vi "Get Hand Info.vi"(10 "Bid":u64, 11 "Hand":string) -> (3 "Hand Info":T1)   [LabVIEW 2023, in "d7.lvlib"]
uses:
  d7.lvlib
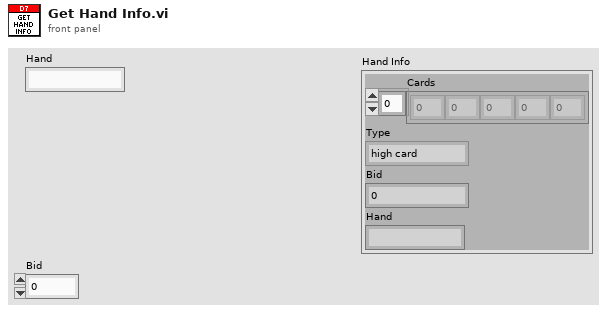
[diagram p1: front panel]
types:
  T1 = cluster{"Cards":i32[], "Type":enum16{"high card", "pair", "two pair", "3 of a kind", "full house", "4 of a kind", "5 of a kind"}, "Bid":u64, "Hand":string}
  T2 = enum16{"high card", "pair", "two pair", "3 of a kind", "full house", "4 of a kind", "5 of a kind"}
  T3 = cluster{i32[], enum16{"high card", "pair", "two pair", "3 of a kind", "full house", "4 of a kind", "5 of a kind"}, "Bid":u64, "Hand":string}
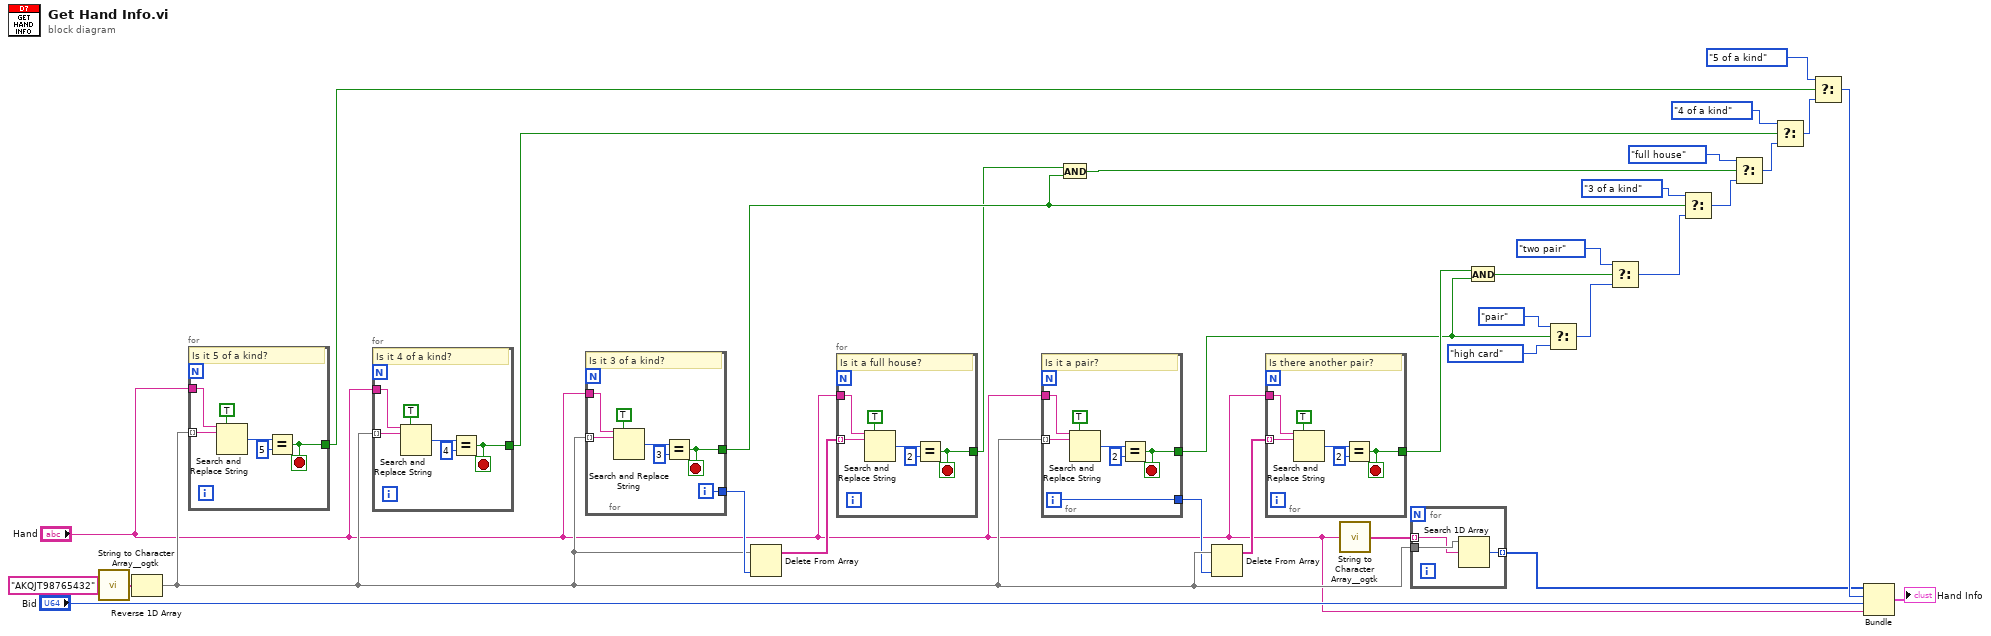
[diagram p0: block diagram]
diagram:
  n1 = call <userlib>:"String to Character Array__ogtk.vi"("Input String"="AKQJT98765432" ("regular expression")) -> ("Character Array"=w17:string[])
  n2 = Reverse 1D Array(array=w17) -> (reversed array=w16:string[])
  n3 = for {
    tunnel: w16 -> [w38] mode=indexing
    tunnel: "Hand" -> [w39]
    tunnel: [w34] -> w31
    stop <- w34 stop-if-true
    # "Is it 5 of a kind?"
    n4 = Search and Replace String(replace all?=TRUE ("replace all? (F)"), input string=w39, search string=w38) -> (number of replacements=w36:i32)  [unwired: 5 in, 3 out]
    n5 = Equal?(x=w36, y=5) -> (x = y?=w34:bool)
  }
  n6 = for {
    tunnel: w16 -> [w44] mode=indexing
    tunnel: "Hand" -> [w45]
    tunnel: [w40] -> w29
    stop <- w40 stop-if-true
    # "Is it 4 of a kind?"
    n7 = Search and Replace String(replace all?=TRUE ("replace all? (F)"), input string=w45, search string=w44) -> (number of replacements=w42:i32)  [unwired: 5 in, 3 out]
    n8 = Equal?(x=w42, y=4) -> (x = y?=w40:bool)
  }
  n9 = for {
    tunnel: w16 -> [w51] mode=indexing
    tunnel: "Hand" -> [w52]
    tunnel: [w47] -> w33
    tunnel: [w46] -> w23
    i -> [w47]
    stop <- w46 stop-if-true
    # "Is it 3 of a kind?"
    n10 = Search and Replace String(replace all?=TRUE ("replace all? (F)"), input string=w52, search string=w51) -> (number of replacements=w49:i32)  [unwired: 5 in, 3 out]
    n11 = Equal?(x=w49, y=3) -> (x = y?=w46:bool)
  }
  n12 = Delete From Array(array=w16, index=w33) -> (array with subset deleted=w32:string[])  [unwired: 1 in, 1 out]
  n13 = for {
    tunnel: w32 -> [w57] mode=indexing
    tunnel: "Hand" -> [w58]
    tunnel: [w53] -> w22
    stop <- w53 stop-if-true
    # "Is it a full house?"
    n14 = Search and Replace String(replace all?=TRUE ("replace all? (F)"), input string=w58, search string=w57) -> (number of replacements=w55:i32)  [unwired: 5 in, 3 out]
    n15 = Equal?(x=w55, y=2) -> (x = y?=w53:bool)
  }
  n16 = for {
    tunnel: w16 -> [w64] mode=indexing
    tunnel: "Hand" -> [w65]
    tunnel: [w60] -> w11
    tunnel: [w59] -> w15
    i -> [w59]
    stop <- w60 stop-if-true
    # "Is it a pair?"
    n17 = Search and Replace String(replace all?=TRUE ("replace all? (F)"), input string=w65, search string=w64) -> (number of replacements=w62:i32)  [unwired: 5 in, 3 out]
    n18 = Equal?(x=w62, y=2) -> (x = y?=w60:bool)
  }
  n19 = And(x=w22, y=w23) -> (x .and. y?=w21:bool)
  n20 = Delete From Array(array=w16, index=w15) -> (array with subset deleted=w14:string[])  [unwired: 1 in, 1 out]
  n21 = for {
    tunnel: w14 -> [w70] mode=indexing
    tunnel: "Hand" -> [w71]
    tunnel: [w66] -> w12
    stop <- w66 stop-if-true
    # "Is there another pair?"
    n22 = Search and Replace String(replace all?=TRUE ("replace all? (F)"), input string=w71, search string=w70) -> (number of replacements=w68:i32)  [unwired: 5 in, 3 out]
    n23 = Equal?(x=w68, y=2) -> (x = y?=w66:bool)
  }
  n24 = call <userlib>:"String to Character Array__ogtk.vi"("Input String"="Hand") -> ("Character Array"=w20:string[])
  n25 = for {
    tunnel: w20 -> [w73] mode=indexing
    tunnel: w16 -> [w74]
    tunnel: [w72] -> w19 mode=indexing
    n26 = Search 1D Array(1D array=w74, element=w73) -> (index of element=w72:i32)  [unwired: 1 in]
  }
  n27 = And(x=w12, y=w11) -> (x .and. y?=w8:bool)
  n28 = Select(t=T2."pair", s=w11, f=T2."high card") -> (s? t:f=w9:T2)
  n29 = Select(t=T2."two pair", s=w8, f=w9) -> (s? t:f=w10:T2)
  n30 = Select(t=T2."3 of a kind", s=w23, f=w10) -> (s? t:f=w27:T2)
  n31 = Select(t=T2."full house", s=w21, f=w27) -> (s? t:f=w28:T2)
  n32 = Select(t=T2."4 of a kind", s=w29, f=w28) -> (s? t:f=w30:T2)
  n33 = Select(t=T2."5 of a kind", s=w31, f=w30) -> (s? t:f=w26:T2)
  n34 = Bundle(w19, w26, "Bid"="Bid", "Hand"="Hand") -> (→"Hand Info":T3)  [unwired: 1 in]
